vi "Line_noAndor.vi"() -> ()   [LabVIEW 2014]
doc: "This is the main user interface of the Raman spectroscopy system."
uses:
  TypeDef/GalvoInput.ctl
  TypeDef/States.ctl
panel:
  in  "Tab Control":enum32{"Main", "Galvo"}(tab)
  in  "Galvo Center":bool
  out "Galvo":bool
  in  "Quit":bool
  out "Initialization finished":bool
  in  "Galvo Stop":bool
  in  "Galvo Scan":bool
  out "CurrentFrame":i32
  in  "Scan parameters":T1={"area/um"=40.7448, "range_x/v"=0.6975, "range_y/v"=0.8477, "interval/um"=0.1598, "x_center/v"=3.35, "y_center/v"=5.55, "theta_1/de"=0.0, "theta_2/de"=60.0, "theta_3/de"=120.0}
  in  "milliseconds to wait":u32=15
  in  "stop":bool
  out "ystep":dbl
  in  "YOffset":dbl=5.55 caption="Offset"
  in  "XOffset":dbl=3.35 caption="Offset"
  out "Sample Rate":dbl=1000.0 format="%0.2f"
  out "Waveform Graph":waveform(dbl)[](graph)=[{"t0"=timestamp(0 s since 1904-01-01), "dt"=0.001, "Y"=[]}]
  in  "ZOffset":dbl=2.0 caption="Offset"
  in  "Galvo":T2={"Sample Rate"=1000000.0, "Sample Clock Source"="OnboardClock", "Max Voltage"=10.0, "Min Voltage"=-10.0, "Physical Channel(s)"="Dev1/ao0,Dev1/ao1,Dev1/ao3"}
  # "Objective: CFI Plan Fluor ELWD 60x (1.27 NA) \nThe depth of field: 1.78 um\nPixel Size: 0.0877um/px"
  # "Galvo Control"
  # "10^4->1s"
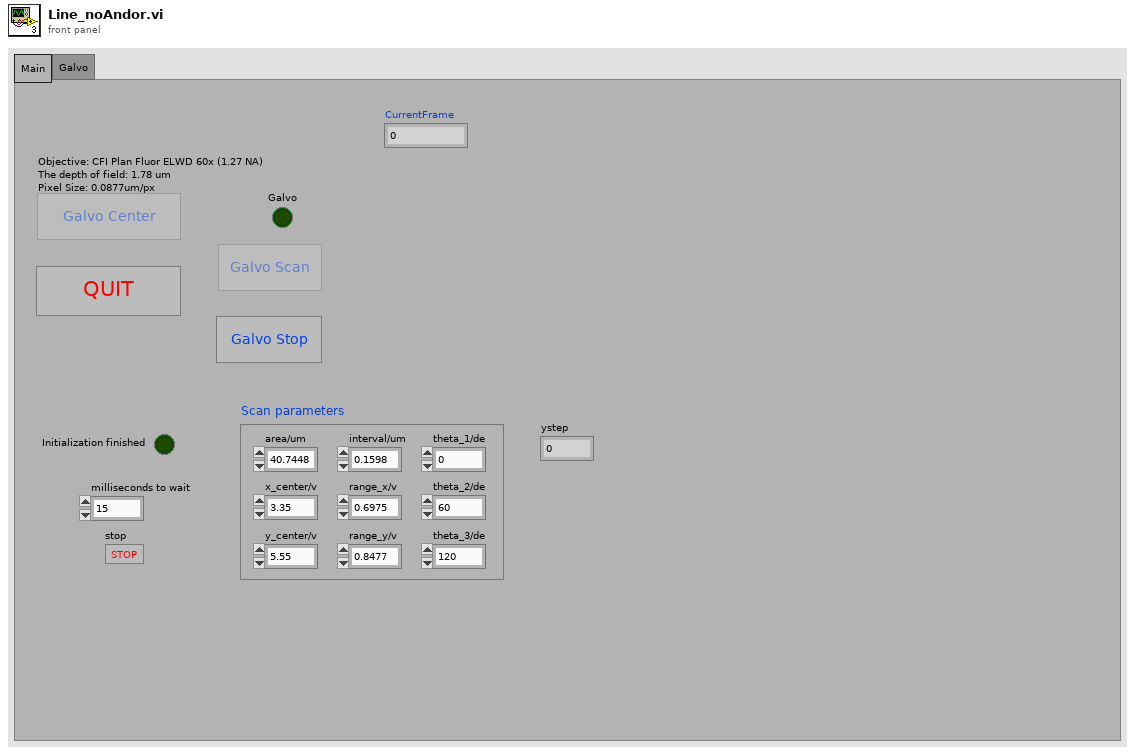
[diagram p1: front panel]
types:
  T1 = cluster{"area/um":dbl, "range_x/v":dbl, "range_y/v":dbl, "interval/um":dbl, "x_center/v":dbl, "y_center/v":dbl, "theta_1/de":dbl, "theta_2/de":dbl, "theta_3/de":dbl}
  T2 = typedef "GalvoInput.ctl" = cluster{"Sample Rate":dbl, "Sample Clock Source":tag, "Max Voltage":dbl, "Min Voltage":dbl, "Physical Channel(s)":tag}
  T3 = typedef "States.ctl" = enum16{"Initialize", "CMOS live", "Shut down"}
  T4 = enum8{"Enabled", "Disabled", "Disabled and Grayed Out"}
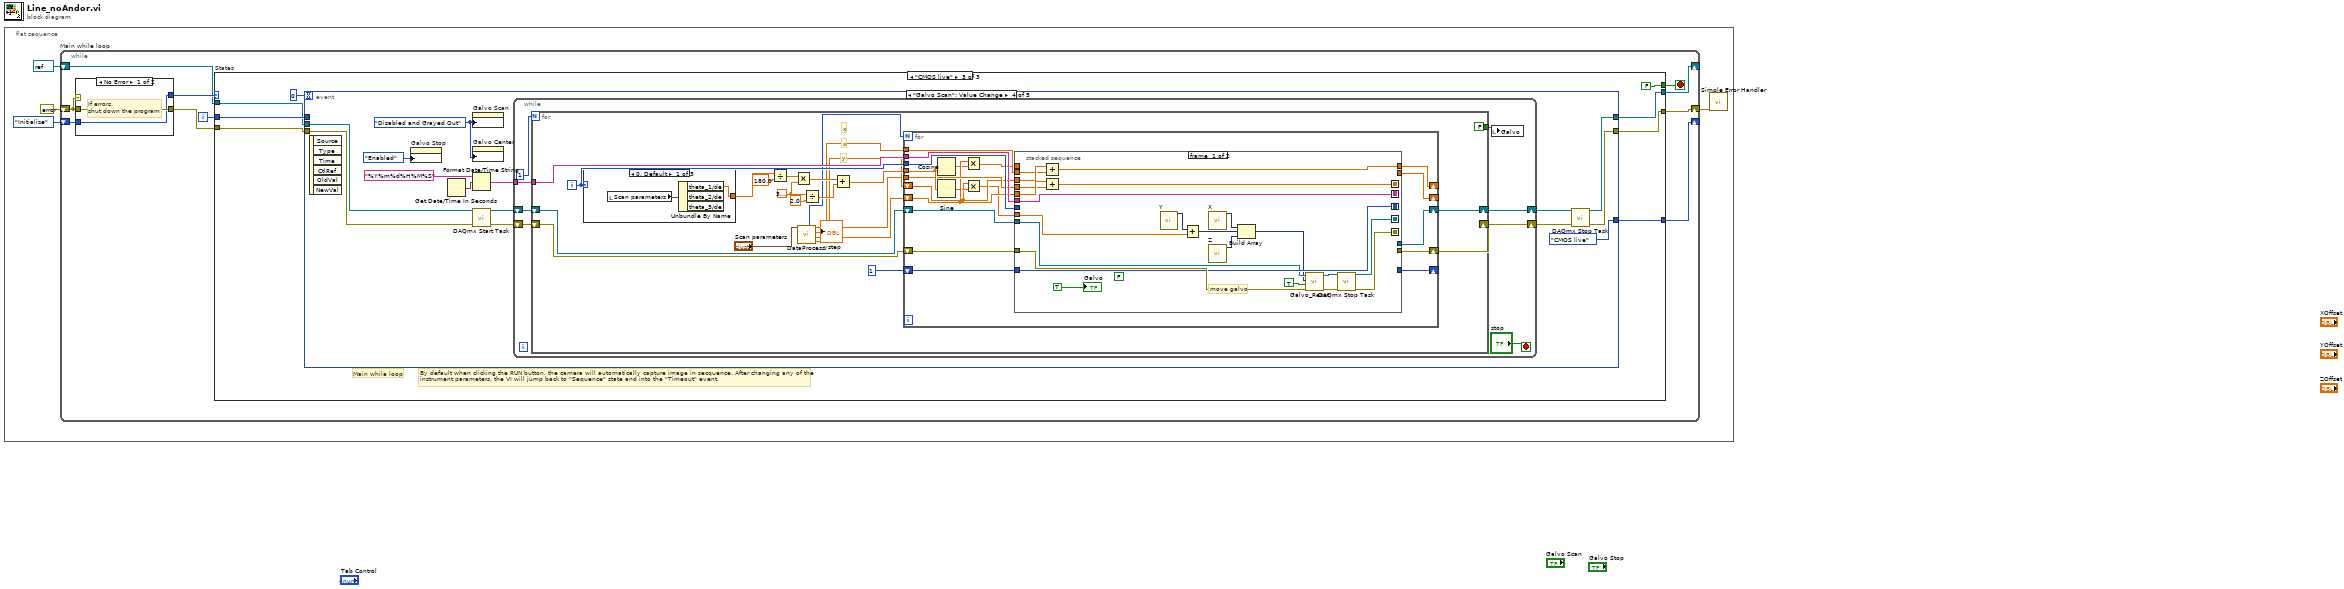
[diagram p0: block diagram]
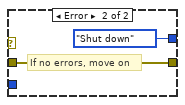
[diagram p2: hidden frame]
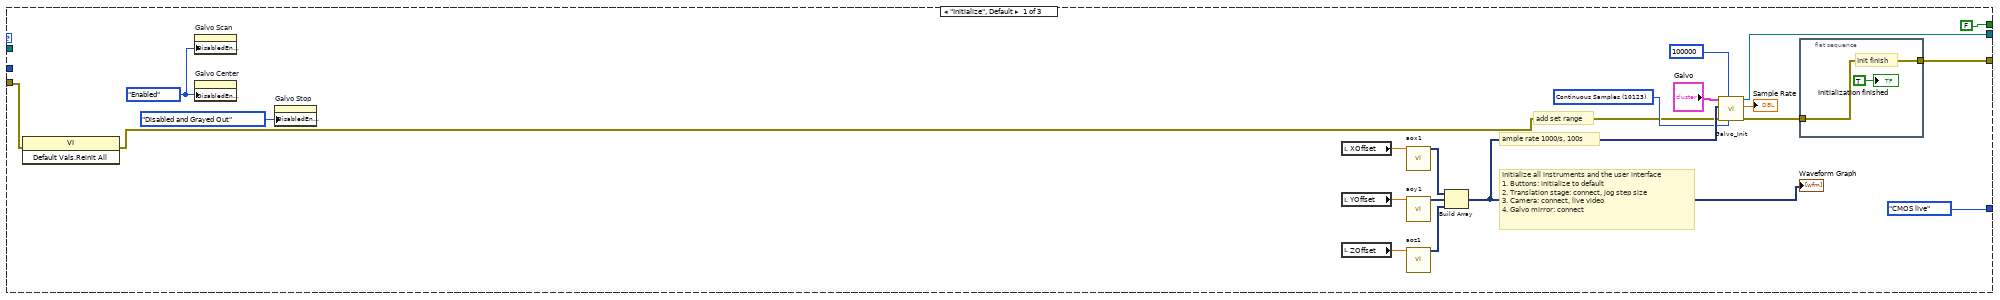
[diagram p3: hidden frame]
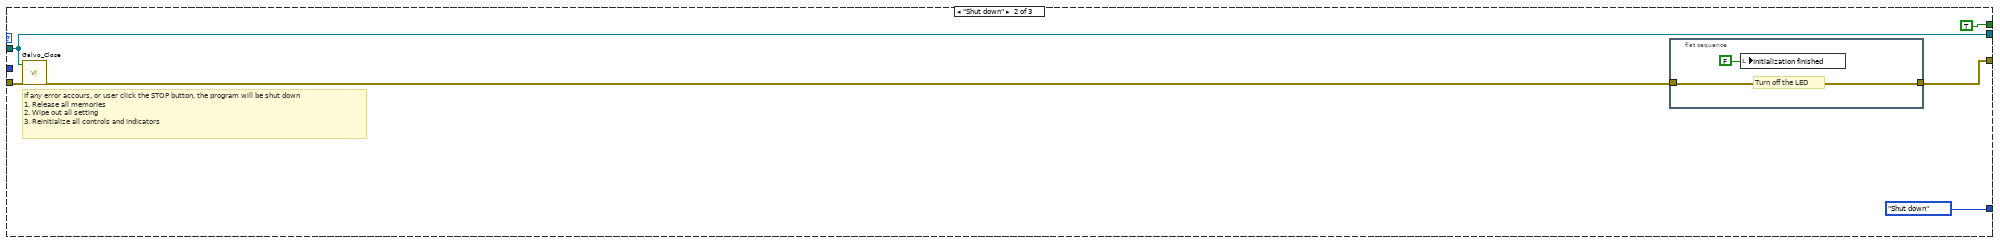
[diagram p4: hidden frame]
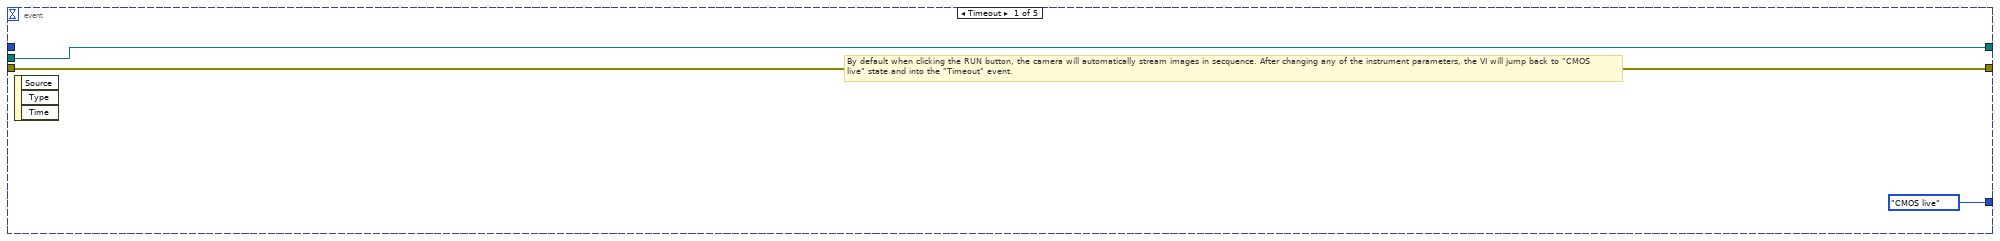
[diagram p5: hidden frame]
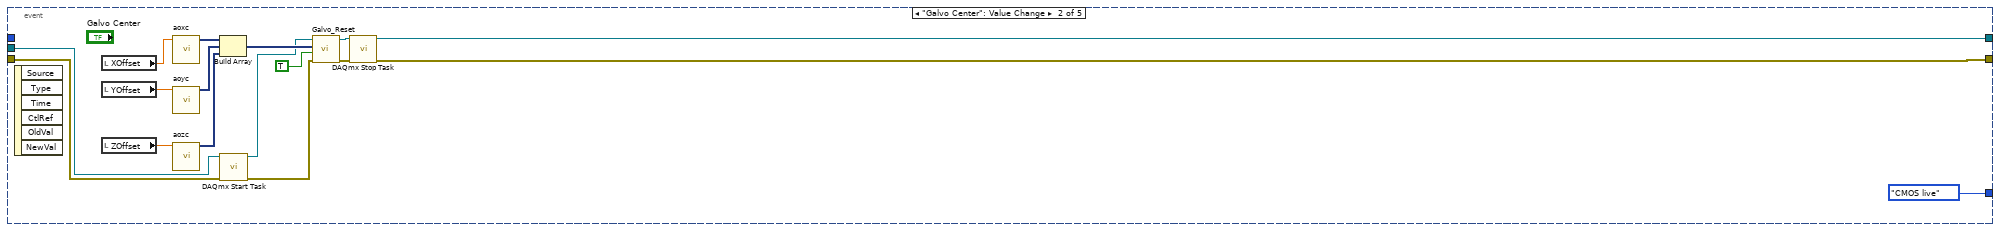
[diagram p6: hidden frame]
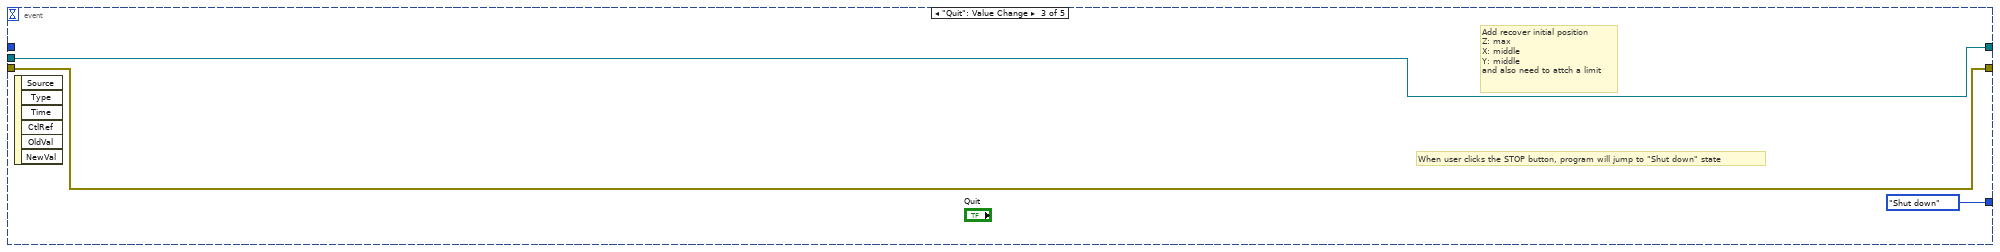
[diagram p7: hidden frame]
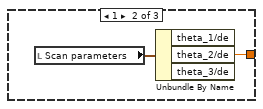
[diagram p8: hidden frame]
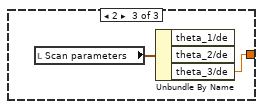
[diagram p9: hidden frame]
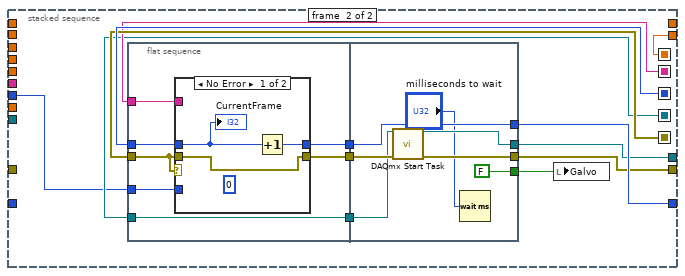
[diagram p10: hidden frame]
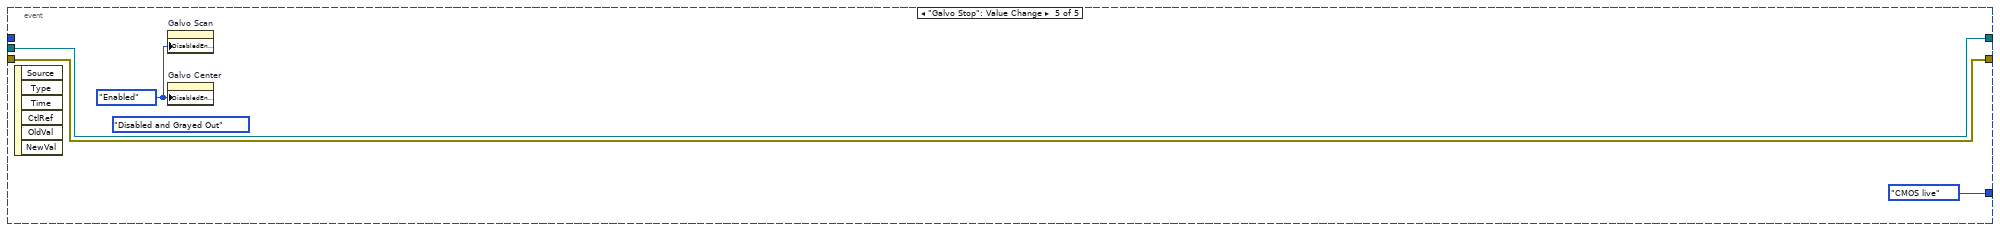
[diagram p12: hidden frame]
diagram:
  n1 = flat-sequence {
    frame #0 {
      n2 = while "Main while loop" {
        shift-right: [w9] -> _
        shift-left: States."Initialize" -> [w14]
        shift-right: [w12] -> w2
        shift-left: errorcluster {"status"=FALSE, "code"=0, "source"=""} ("error out") -> [w8]
        shift-right: [w6] -> _
        shift-left: refnum<k21> refnum ("task out") -> [w5]
        i -> [w7]
        stop <- w10 stop-if-true
        n3 = case shown="No Error" w8 {
          tunnel: w8 -> [w16 w18]
          tunnel: [w16 w18] -> w11
          tunnel: w14 -> [w15 _]
          tunnel: [w15 States."Shut down"] -> w13
          frame No Error {
            # "If errors,\nshut down the program"
          }
          frame Error {
            # "If no errors, move on"
          }
        }
        n4 = case "States" shown="\"CMOS live\"" w13 {
          tunnel: [w36 w41 w54] -> w12
          tunnel: w11 -> [w37 w42 w55]
          tunnel: [FALSE TRUE FALSE] -> w10
          tunnel: [States."CMOS live" States."Shut down" w56] -> w9
          tunnel: w7 -> [_ _ w52]
          tunnel: [w33 w44 w50] -> w6
          tunnel: w5 -> [_ w44 w51]
          frame "Initialize", Default {
            w22 = T4."Enabled" ("Disabled")
            w28 = 10123 items=["Finite Samples"=10178, "Continuous Samples"=10123, "Hardware Timed Single Point"=12522] ("Sample Mode")
            # "ample rate 1000/s, 100s"
            # "add set range"
            # "Initialize all instruments and the user interface\n1. Buttons: initialize to default\n2. Translation stage: connect, jog step size\n3. Camera: connect, live video\n4. Galvo mirror: connect"
            n5 = invoke class="VI" method="Default Vals.Reinit All"(error in=w37) -> (error out=w21:errorcluster)  [unwired: 2 in, 2 out]
            n6 = property on="Galvo Scan" class="Bool"("DisabledEnum"=w22) -> ()  [unwired: 2 in, 2 out]
            n7 = property on="Galvo Center" class="Bool"("DisabledEnum"=w22) -> ()  [unwired: 2 in, 2 out]
            n8 = property on="Galvo Stop" class="Bool"("DisabledEnum"=T4."Disabled and Grayed Out" ("Disabled")) -> ()  [unwired: 2 in, 2 out]
            n9 = local read "XOffset"() -> (w25:dbl)
            n10 = local read "YOffset"() -> (w24:dbl)
            n11 = local read "ZOffset"() -> (w23:dbl)
            n12 = call "aox1"("Offset"=w25) -> ("DC"=w27:dynamicdata)  [unwired: 13 in, 1 out]
            n13 = call "aoy1"("Offset"=w24) -> ("DC"=w26:dynamicdata)  [unwired: 13 in, 1 out]
            n14 = call "aoz1"("Offset"=w23) -> ("DC"=w31:dynamicdata)  [unwired: 13 in, 1 out]
            n15 = Build Array(w27, w26, w31) -> (w30:dynamicdata[])
            "Waveform Graph" <- w30
            n16 = call "Galvo_Init.vi"("Sample Mode"=w28, "samples per channel"=100000, "error in"=w21, "Signal array"=w30, "Galvo_Input"="Galvo") -> ("error out"=w32:errorcluster, "Actual Sample Rate"=→"Sample Rate":dbl, "task out"=w33:refnum<k21>)  [unwired: 4 in]
            n17 = flat-sequence {
              tunnel: w32 -> [w40]
              tunnel: [w40] -> w36
              frame #0 {
                # "Init finish"
                "Initialization finished" <- TRUE ("Initialization finished")
              }
            }
          }
          frame "Shut down" {
            # "If any error accours, or user click the STOP button, the program will be shut down\n1. Release all memories\n2. Wipe out all setting\n3. Reinitialize all controls and indicators"
            n18 = call "Galvo_Close.vi"("error in"=w42, "task/channels in"=w44) -> ("error out"=w43:errorcluster)  [unwired: 9 in]
            n19 = flat-sequence {
              tunnel: w43 -> [w47]
              tunnel: [w47] -> w41
              frame #0 {
                # "Turn off the LED"
                n20 = local write "Initialization finished"(FALSE ("Initialization finished")) -> ()
              }
            }
          }
          frame "CMOS live" {
            # "Main while loop"
            # "By default when clicking the RUN button, the camera will automatically capture image in secquence. After changing any of the \ninstrument parameters, the VI will jump back to \"Sequence\" state and into the \"Timeout\" event."
            n21 = event shown="[3] \"Galvo Scan\": Value Change" {
              selector: _ -> [_ _ _ _ _]
              dyn-events: _ -> [_ _ _ _ _]
              timeout: 0 -> [_ _ _ _ _]
              tunnel: [States."CMOS live" States."CMOS live" States."Shut down" States."CMOS live" States."CMOS live"] -> w56
              tunnel: w55 -> [w57 w68 w78 w82 w203]
              tunnel: [w57 w62 w78 w87 w203] -> w54
              tunnel: w52 -> [_ _ _ _ _]
              tunnel: [w59 w63 w77 w86 w205] -> w50
              tunnel: w51 -> [w59 w70 w77 w92 w205]
              event Timeout {
                # "By default when clicking the RUN button, the camera will automatically stream images in secquence. After changing any of the instrument parameters, the VI will jump back to \"CMOS live\" state and into the \"Timeout\" event."
                n22 = event-data() -> ()  [unwired: 1 in, 3 out]
              }
              event "Galvo Center": Value Change {
                n23 = event-data() -> ()  [unwired: 1 in, 6 out]
                n24 = local read "XOffset"() -> (w61:dbl)
                n25 = local read "YOffset"() -> (w60:dbl)
                n26 = local read "ZOffset"() -> (w74:dbl)
                n27 = call "aoxc"("Offset"=w61) -> ("DC"=w72:dynamicdata)  [unwired: 13 in, 1 out]
                n28 = call "aoyc"("Offset"=w60) -> ("DC"=w71:dynamicdata)  [unwired: 13 in, 1 out]
                n29 = call "aozc"("Offset"=w74) -> ("DC"=w75:dynamicdata)  [unwired: 13 in, 1 out]
                n30 = Build Array(w72, w71, w75) -> (w73:dynamicdata[])
                n31 = call <vilib>:"DAQmx Start Task.vi"("task/channels in"=w70, "error in"=w68) -> ("task out"=w69:refnum<k21>, "error out"=w67:errorcluster)  [unwired: 12 in]
                n32 = call "Galvo_Reset.vi"("error in"=w67, "auto start"=TRUE, "Signal array"=w73, "task/channels in"=w69) -> ("error out"=w64:errorcluster, "task out"=w65:refnum<k21>)  [unwired: 6 in]
                n33 = call <vilib>:"DAQmx Stop Task.vi"("task/channels in"=w65, "error in"=w64) -> ("task out"=w63:refnum<k21>, "error out"=w62:errorcluster)  [unwired: 12 in]
              }
              event "Quit": Value Change {
                # "Add recover initial position\nZ: max\nX: middle\nY: middle\nand also need to attch a limit"
                # "When user clicks the STOP button, program will jump to \"Shut down\" state"
                n34 = event-data() -> ()  [unwired: 1 in, 6 out]
              }
              event "Galvo Scan": Value Change {
                w80 = T4."Disabled and Grayed Out" ("Disabled")
                n35 = event-data() -> ()  [unwired: 1 in, 6 out]
                n36 = property on="Galvo Stop" class="Bool"("DisabledEnum"=T4."Enabled" ("Disabled")) -> ()  [unwired: 2 in, 2 out]
                n37 = Get Date/Time In Seconds() -> (seconds since 1Jan1904=w85:timestamp)
                n38 = property on="Galvo Scan" class="Bool"("DisabledEnum"=w80) -> ()  [unwired: 2 in, 2 out]
                n39 = property on="Galvo Center" class="Bool"("DisabledEnum"=w80) -> ()  [unwired: 2 in, 2 out]
                n40 = Format Date/Time String(time format string (%c)="%Y%m%d%H%M%S", seconds (now)=w85) -> (date/time string=w83:string)  [unwired: 1 in]
                n41 = call <vilib>:"DAQmx Start Task.vi"("task/channels in"=w92, "error in"=w82) -> ("task out"=w90:refnum<k21>, "error out"=w91:errorcluster)  [unwired: 12 in]
                n42 = while {
                  tunnel: w83 -> [w96]
                  shift-right: [w97] -> w88
                  shift-left: w91 -> [w101]
                  shift-right: [w98] -> w89
                  shift-left: w90 -> [w99]
                  stop <- "stop" stop-if-true
                  n43 = for {
                    N: 1 -> [_]
                    tunnel: [FALSE ("Galvo")] -> w100
                    shift-right: [w122] -> w97
                    shift-left: w101 -> [w121]
                    shift-right: [w119] -> w98
                    shift-left: w99 -> [w120]
                    tunnel: w96 -> [w118]
                    i -> [w109]
                    w113 = 3.141592653589793
                    # "y"
                    # "x"
                    # "x"
                    n44 = case shown="0, Default" w109 {
                      tunnel: [w124 w126 w128] -> w116
                      frame 0, Default {
                        n45 = local read "Scan parameters"() -> (w125:T1)
                        n46 = Unbundle By Name(w125) -> ("theta_1/de"=w124:dbl)  [unwired: 2 out]
                      }
                      frame 1 {
                        n47 = local read "Scan parameters"() -> (w127:T1)
                        n48 = Unbundle By Name(w127) -> ("theta_2/de"=w126:dbl)  [unwired: 2 out]
                      }
                      frame 2 {
                        n49 = local read "Scan parameters"() -> (w129:T1)
                        n50 = Unbundle By Name(w129) -> ("theta_3/de"=w128:dbl)  [unwired: 2 out]
                      }
                    }
                    n51 = Divide(x=w116, y=180.0 ("x")) -> (x/y=w115:dbl)
                    n52 = Multiply(x=w115, y=w113) -> (x*y=w114:dbl)
                    n53 = call "DataProcess.vi"("Scan parameters"="Scan parameters") -> ("ystart"=w104:dbl, "xstart"=w105:dbl, "ystep"=w102:dbl, "xstep"=w103:dbl, "NUM"=w106:i32)  [unwired: 6 in]
                    "ystep" <- w102
                    n54 = Divide(x=w113, y=2.0) -> (x/y=w112:dbl)
                    n55 = Add(x=w114, y=w112) -> (x+y=w110:dbl)
                    n56 = for {
                      N: w106 -> [_]
                      shift-right: [w143] -> w122
                      shift-left: w121 -> [w148]
                      shift-right: [w144] -> w119
                      shift-left: w120 -> [w147]
                      shift-right: [w142] -> _
                      shift-left: 1 -> [w146]
                      tunnel: w118 -> [w145]
                      tunnel: w110 -> [w141]
                      shift-right: [w138] -> _
                      shift-left: w105 -> [w135]
                      shift-right: [w139] -> _
                      shift-left: w104 -> [w132]
                      tunnel: w109 -> [w140]
                      tunnel: w103 -> [w137]
                      tunnel: w102 -> [w136]
                      n57 = Cosine(x=w141) -> (cos(x)=w134:dbl)
                      n58 = Sine(x=w141) -> (sin(x)=w133:dbl)
                      n59 = Multiply(x=w135, y=w134) -> (x*y=w130:dbl)
                      n60 = Multiply(x=w132, y=w133) -> (x*y=w131:dbl)
                      n61 = stacked-sequence {
                        seq-local: [w166 _] -> [_ w176]
                        seq-local: [w168 _] -> [_ w177]
                        seq-local: [w164 _] -> [_ w182]
                        seq-local: [w163 _] -> [_ w175]
                        seq-local: [w160 _] -> [_ w174]
                        tunnel: w148 -> [w169 _]
                        tunnel: w147 -> [w162 _]
                        tunnel: w146 -> [w164 _]
                        tunnel: w145 -> [w163 _]
                        tunnel: [_ w177] -> w138
                        tunnel: [_ w180] -> w142
                        tunnel: [_ w179] -> w143
                        tunnel: [_ w172] -> w144
                        tunnel: w130 -> [_ _]
                        tunnel: w131 -> [w153 _]
                        tunnel: w135 -> [w157 _]
                        tunnel: w132 -> [w156 _]
                        tunnel: [w155 _] -> w139
                        tunnel: w140 -> [_ w171]
                        tunnel: w137 -> [w152 _]
                        tunnel: w136 -> [w151 _]
                        frame #0 {
                          (unwired) FALSE ("SaveStatus")
                          # "move galvo"
                          n62 = Add(x=w156, y=w151) -> (x+y=w155:dbl)
                          n63 = Add(x=w157, y=w152) -> (x+y=w168:dbl)
                          n64 = call "Y"() -> ("Signal"=w158:dynamicdata)  [unwired: 9 in, 2 out]
                          n65 = Add(x=w158, y=w153) -> (x+y=w159:dynamicdata)
                          n66 = call "X"() -> ("Signal"=w149:dynamicdata)  [unwired: 9 in, 2 out]
                          n67 = call "Z"() -> ("Signal"=w154:dynamicdata)  [unwired: 9 in, 2 out]
                          n68 = Build Array(w149, w159, w154) -> (w150:dynamicdata[])
                          n69 = call "Galvo_Reset.vi"("error in"=w169, "auto start"=TRUE, "Signal array"=w150, "task/channels in"=w162) -> ("error out"=w167:errorcluster, "task out"=w161:refnum<k21>)  [unwired: 6 in]
                          n70 = call <vilib>:"DAQmx Stop Task.vi"("task/channels in"=w161, "error in"=w167) -> ("task out"=w160:refnum<k21>, "error out"=w166:errorcluster)  [unwired: 12 in]
                          "Galvo" <- TRUE
                        }
                        frame #1 {
                          n71 = flat-sequence {
                            tunnel: [w190] -> w183
                            tunnel: w182 -> [w189]
                            tunnel: [w188] -> w181
                            tunnel: w176 -> [w187]
                            tunnel: w175 -> [w186]
                            tunnel: w174 -> [w185]
                            tunnel: [w185] -> w173
                            tunnel: w171 -> [w184]
                            tunnel: [w197] -> w179
                            tunnel: w183 -> [w201]
                            tunnel: w181 -> [w202]
                            tunnel: [w202] -> w180
                            tunnel: [FALSE ("Galvo")] -> w178
                            tunnel: w173 -> [w199]
                            tunnel: [w198] -> w172
                            frame #0 {
                              n72 = case shown="No Error" w187 {
                                tunnel: [w191 w194] -> w190
                                tunnel: [w193 w195] -> w188
                                tunnel: w189 -> [w192 w195]
                                tunnel: w187 -> [w191 w194]
                                tunnel: w186 -> [_ _]
                                tunnel: w184 -> [_ _]
                                frame No Error {
                                (unwired) 0 ("Phase")
                                n73 = Increment(x=w192) -> (x+1=w193:i32)
                                "CurrentFrame" <- w192
                                }
                                frame Error {
                                }
                              }
                            }
                            frame #1 {
                              n74 = call <vilib>:"DAQmx Start Task.vi"("task/channels in"=w199, "error in"=w201) -> ("task out"=w198:refnum<k21>, "error out"=w197:errorcluster)  [unwired: 12 in]
                              n75 = Wait (ms)(milliseconds to wait="milliseconds to wait") -> ()  [unwired: 1 out]
                            }
                          }
                          n76 = local write "Galvo"(w178) -> ()
                        }
                      }
                    }
                  }
                  n77 = local write "Galvo"(w100) -> ()
                }
                n78 = call <vilib>:"DAQmx Stop Task.vi"("task/channels in"=w89, "error in"=w88) -> ("task out"=w86:refnum<k21>, "error out"=w87:errorcluster)  [unwired: 12 in]
              }
              event "Galvo Stop": Value Change {
                (unwired) T4."Disabled and Grayed Out" ("Disabled")
                w204 = T4."Enabled" ("Disabled")
                n79 = event-data() -> ()  [unwired: 1 in, 6 out]
                n80 = property on="Galvo Scan" class="Bool"("DisabledEnum"=w204) -> ()  [unwired: 2 in, 2 out]
                n81 = property on="Galvo Center" class="Bool"("DisabledEnum"=w204) -> ()  [unwired: 2 in, 2 out]
              }
            }
          }
        }
      }
      n82 = call <vilib>:"Simple Error Handler.vi"("error in (no error)"=w2) -> ()  [unwired: 4 in, 5 out]
    }
  }
